vi "Set Close Log after Trigger.vi"(8 "error in (no error)":errorcluster, 10 "Close Log after Trigger":bool, 11 "Triggered Log in":refnum<class "Triggered Log.lvclass">) -> (0 "error out":errorcluster, 3 "Triggered Log out":refnum<class "Triggered Log.lvclass">)   [LabVIEW 2012, in "Triggered Log.lvclass"]
uses:
  Triggered Log.lvclass
  Triggered Log.lvclass/Triggered Log.ctl
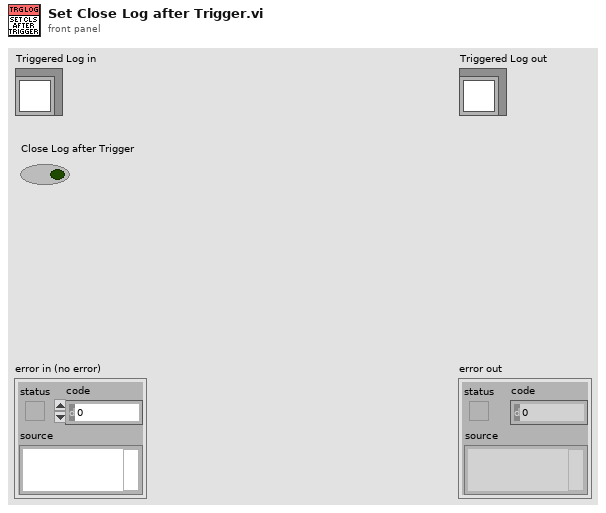
[diagram p1: front panel]
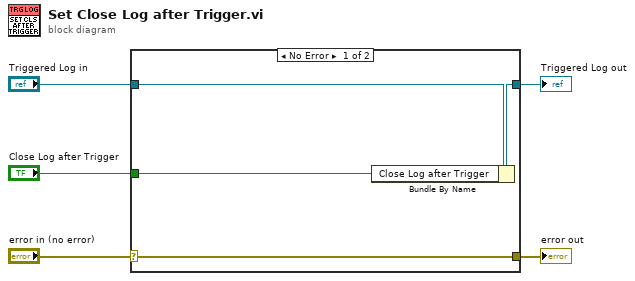
[diagram p0: block diagram]
diagram:
  n1 = case shown="No Error" "error in (no error)" {
    selector: "error in (no error)" -> [w9 w10]
    tunnel: [w9 w10] -> w4
    tunnel: [w7 w11] -> w2
    tunnel: "Triggered Log in" -> [w8 w11]
    tunnel: "Close Log after Trigger" -> [w6 _]
    frame No Error {
      n2 = Bundle By Name(cluster=w8, "Close Log after Trigger"=w6) -> (w7:refnum<class "Triggered Log.lvclass">)
    }
    frame Error {
    }
  }
  "error out" <- w4
  "Triggered Log out" <- w2
